vi "Read Name.vi"(8 "error in":errorcluster, 11 "Engine in":refnum<class "Engine Parent Editor Node.lvclass">) -> (0 "error out":errorcluster, 2 "Name":string, 3 "Engine out":refnum<class "Engine Parent Editor Node.lvclass">)   [LabVIEW 2013, in "PL Framework Configuration Tool.lvlib" / "Engine Parent Editor Node.lvclass"]
uses:
  Engine Parent Editor Node.lvclass
  <vilib>/NI/Configuration Framework/serializable configuration/NISE_CEF_serializable configuration.lvclass
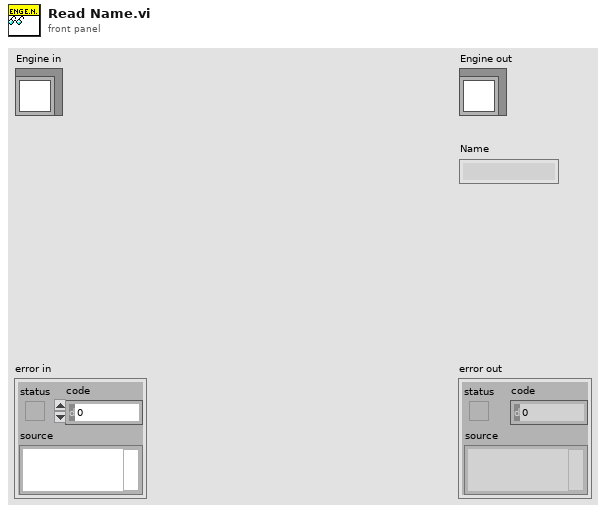
[diagram p1: front panel]
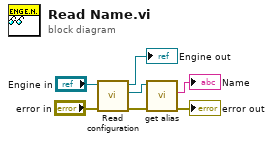
[diagram p0: block diagram]
diagram:
  n1 = call-dynamic "Read configuration.vi"("error in"="error in", "NISE_CEF_serializable node in"="Engine in") -> ("error out"=w4:errorcluster, "configuration"=w3:refnum<class "NISE_CEF_serializable configuration.lvclass">, "NISE_CEF_serializable node out"=→"Engine out":refnum<class "Engine Parent Editor Node.lvclass">)  [unwired: 7 in]
  n2 = call <vilib>:"get alias.vi"("error in"=w4, "configuration in"=w3) -> ("error out"=→"error out":errorcluster, "alias"=→"Name":string)  [unwired: 7 in, 1 out]
